vi "output.vi"(8 "error in":errorcluster, 10 "data table in":T1, 11 "dds runtime in":refnum<class "dds runtime.lvclass">) -> (0 "error out":errorcluster, 2 "data table out":T1, 3 "dds runtime out":refnum<class "dds runtime.lvclass">)   [LabVIEW 2015, in "DDS runtime.lvclass"]
doc: "Provides an interface for writing data to a module at runtime. While this interface performs no operations, a child should provide an override which may write to any open sessions, references, or interfaces."
uses:
  DDS runtime.lvclass
  <vilib>/NI/Tag Bus/table/data table.ctl
  DDS runtime.lvclass/dds runtime.ctl
  <vilib>/NI/Tag Bus/table/data polymorphs/read one/read Double.vi
  <vilib>/RTI DDS Toolkit/VIs/Write_Num.vi
  <vilib>/NI/Tag Bus/table/data polymorphs/read one/read Single.vi
  <vilib>/RTI DDS Toolkit/VIs/Write_NumSgl.vi
  <vilib>/NI/Tag Bus/table/data polymorphs/read one/read I64.vi
  <vilib>/RTI DDS Toolkit/VIs/Write_NumI64.vi
  <vilib>/NI/Tag Bus/table/data polymorphs/read one/read I32.vi
  <vilib>/RTI DDS Toolkit/VIs/Write_NumI32.vi
  <vilib>/NI/Tag Bus/table/data polymorphs/read one/read I16.vi
  <vilib>/RTI DDS Toolkit/VIs/Write_NumI16.vi
  <vilib>/NI/Tag Bus/table/data polymorphs/read one/read I8.vi
  <vilib>/RTI DDS Toolkit/VIs/Write_NumI8.vi
  <vilib>/NI/Tag Bus/table/data polymorphs/read one/read U64.vi
  <vilib>/RTI DDS Toolkit/VIs/Write_NumU64.vi
  <vilib>/NI/Tag Bus/table/data polymorphs/read one/read U32.vi
  <vilib>/RTI DDS Toolkit/VIs/Write_NumU32.vi
  <vilib>/NI/Tag Bus/table/data polymorphs/read one/read U16.vi
  <vilib>/RTI DDS Toolkit/VIs/Write_NumU16.vi
  <vilib>/NI/Tag Bus/table/data polymorphs/read one/read U8.vi
  <vilib>/RTI DDS Toolkit/VIs/Write_NumU8.vi
  <vilib>/NI/Tag Bus/table/data polymorphs/read one/read Boolean.vi
  <vilib>/RTI DDS Toolkit/VIs/Write_Bool.vi
  <vilib>/NI/Tag Bus/table/data polymorphs/read one/read String.vi
  <vilib>/RTI DDS Toolkit/VIs/Write_String.vi
  <vilib>/RTI DDS Toolkit/Library/LVDDS_library.lvlib
  <vilib>/NI/Tag Bus/table/data table.lvlib
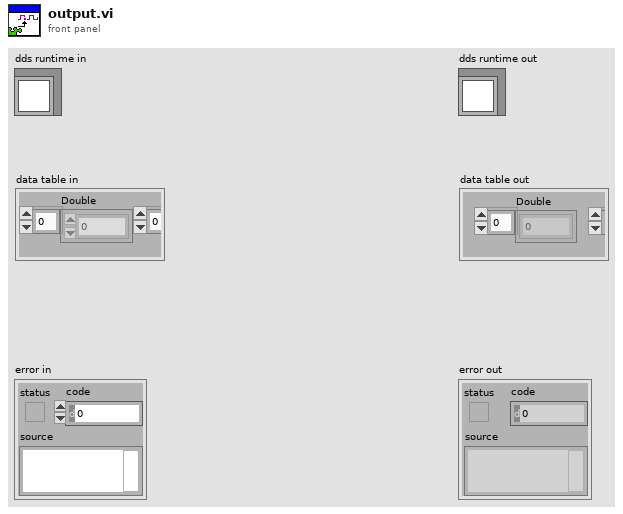
[diagram p1: front panel]
types:
  T1 = typedef "tag bus.lvlib/data table.lvlib/data table.ctl" = cluster{"Double":dbl[], "Single":sgl[], "I64":i64[], "I32":i32[], "I16":i16[], "I8":i8[], "U64":u64[], "U32":u32[], "U16":u16[], "U8":u8[], "Boolean":bool[], "String":string[], "Array of Double":cluster{"DBL Array":dbl[]}[], "Array of Single":cluster{"SGL Array":sgl[]}[], "Array of I64":cluster{"I64 Array":i64[]}[], "Array of I32":cluster{"I32 Array":i32[]}[], "Array of I16":cluster{"I16 Array":i16[]}[], "Array of I8":cluster{"I8 Array":i8[]}[], "Array of U64":cluster{"U64 Array":u64[]}[], "Array of U32":cluster{"U32 Array":u32[]}[], "Array of U16":cluster{"U16 Array":u16[]}[], "Array of U8":cluster{"U8 Array":u8[]}[], "Array of Boolean":cluster{"Boolean Array":bool[]}[], "Array of String":cluster{"String Array":string[]}[]}
  T2 = typedef "tag bus.lvlib/tag descriptor.lvclass/Data Type.ctl" = enum16{"Double", "Single", "I64", "I32", "I16", "I8", "U64", "U32", "U16", "U8", "Boolean", "String", "Array of Double", "Array of Single", "Array of I64", "Array of I32", "Array of I16", "Array of I8", "Array of U64", "Array of U32", "Array of U16", "Array of U8", "Array of Boolean", "Array of String"}
  T3 = cluster{"index":i32, "data type":T2, "ref num":u64}[]
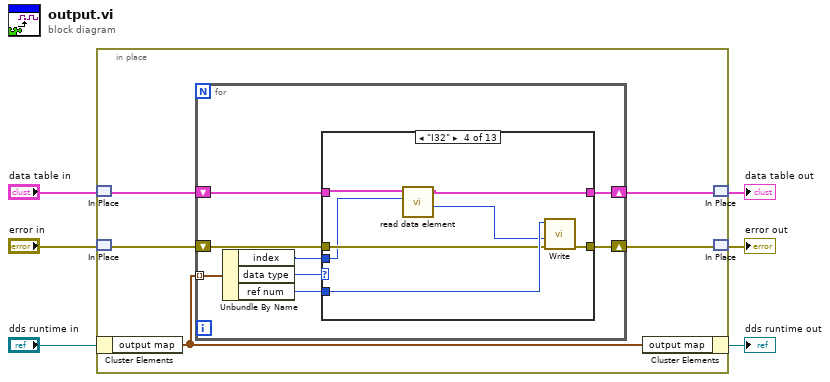
[diagram p0: block diagram]
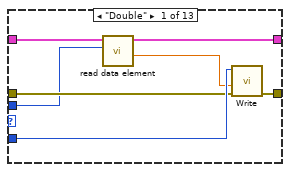
[diagram p2: hidden frame]
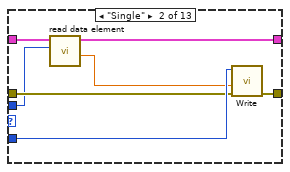
[diagram p3: hidden frame]
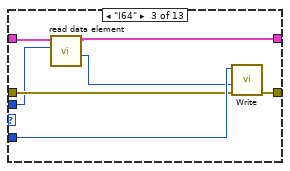
[diagram p4: hidden frame]
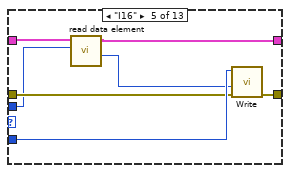
[diagram p5: hidden frame]
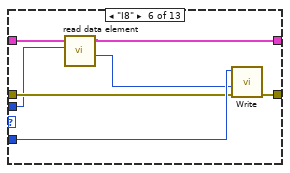
[diagram p6: hidden frame]
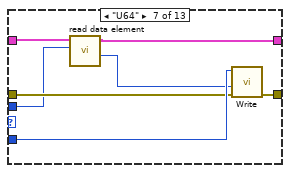
[diagram p7: hidden frame]
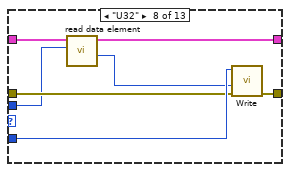
[diagram p8: hidden frame]
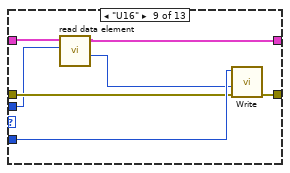
[diagram p9: hidden frame]
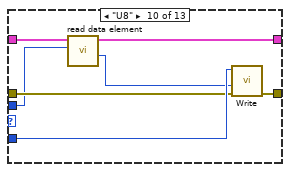
[diagram p10: hidden frame]
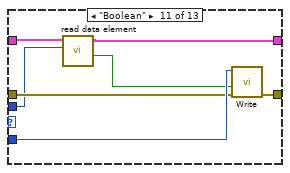
[diagram p11: hidden frame]
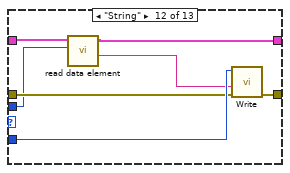
[diagram p12: hidden frame]
diagram:
  n1 = in-place {
    n2 = in-place-match #1("data table in") -> (w11:T1)
    n3 = in-place-match #2("error in") -> (w10:errorcluster)
    n4 = in-place-cluster #3("dds runtime in") -> ("output map"=w7:T3)
    n5 = for {
      tunnel: w7 -> [w19] mode=indexing
      shift-right: [w13] -> w8
      shift-left: w11 -> [w18]
      shift-right: [w14] -> w9
      shift-left: w10 -> [w15]
      n6 = Unbundle By Name(w19) -> ("index"=w17:i32, "data type"=w12:T2, "ref num"=w16:u64)
      n7 = case shown="\"I32\"" w12 {
        tunnel: w18 -> [w21 w30 w37 w44 w51 w58 w65 w72 w78 w86 w93 w100 w105]
        tunnel: w17 -> [w20 w28 w35 w41 w48 w56 w62 w69 w77 w83 w90 w98 _]
        tunnel: w16 -> [w26 w33 w40 w47 w54 w61 w68 w75 w82 w89 w96 w103 _]
        tunnel: w15 -> [w24 w32 w39 w46 w53 w60 w67 w74 w81 w88 w95 w102 w104]
        tunnel: [w23 w31 w38 w45 w52 w59 w66 w73 w80 w87 w94 w101 w104] -> w14
        tunnel: [w22 w29 w36 w43 w50 w57 w64 w71 w79 w85 w92 w99 w105] -> w13
        frame "Double" {
          n8 = call-poly <vilib>:"read data element.vi"("index"=w20, "data table in"=w21) -> ("value"=w25:dbl, "data table out"=w22:T1)  [unwired: 8 in]
          n9 = call-poly <vilib>:"Write.vi"("error in (no error)"=w24, "Data"=w25, "DDS Object Ref in"=w26) -> ("error out"=w23:errorcluster)  [unwired: 7 in, 1 out]
        }
        frame "Single" {
          n10 = call-poly <vilib>:"read data element.vi"("index"=w28, "data table in"=w30) -> ("value"=w27:sgl, "data table out"=w29:T1)  [unwired: 8 in]
          n11 = call-poly <vilib>:"Write.vi"("error in (no error)"=w32, "Data"=w27, "DDS Object Ref in"=w33) -> ("error out"=w31:errorcluster)  [unwired: 7 in, 1 out]
        }
        frame "I64" {
          n12 = call-poly <vilib>:"read data element.vi"("index"=w35, "data table in"=w37) -> ("value"=w34:i64, "data table out"=w36:T1)  [unwired: 8 in]
          n13 = call-poly <vilib>:"Write.vi"("error in (no error)"=w39, "Data"=w34, "DDS Object Ref in"=w40) -> ("error out"=w38:errorcluster)  [unwired: 7 in, 1 out]
        }
        frame "I32" {
          n14 = call-poly <vilib>:"read data element.vi"("index"=w41, "data table in"=w44) -> ("value"=w42:i32, "data table out"=w43:T1)  [unwired: 8 in]
          n15 = call-poly <vilib>:"Write.vi"("error in (no error)"=w46, "Data"=w42, "DDS Object Ref in"=w47) -> ("error out"=w45:errorcluster)  [unwired: 7 in, 1 out]
        }
        frame "I16" {
          n16 = call-poly <vilib>:"read data element.vi"("index"=w48, "data table in"=w51) -> ("value"=w49:i16, "data table out"=w50:T1)  [unwired: 8 in]
          n17 = call-poly <vilib>:"Write.vi"("error in (no error)"=w53, "Data"=w49, "DDS Object Ref in"=w54) -> ("error out"=w52:errorcluster)  [unwired: 7 in, 1 out]
        }
        frame "I8" {
          n18 = call-poly <vilib>:"read data element.vi"("index"=w56, "data table in"=w58) -> ("value"=w55:i8, "data table out"=w57:T1)  [unwired: 8 in]
          n19 = call-poly <vilib>:"Write.vi"("error in (no error)"=w60, "Data"=w55, "DDS Object Ref in"=w61) -> ("error out"=w59:errorcluster)  [unwired: 7 in, 1 out]
        }
        frame "U64" {
          n20 = call-poly <vilib>:"read data element.vi"("index"=w62, "data table in"=w65) -> ("value"=w63:u64, "data table out"=w64:T1)  [unwired: 8 in]
          n21 = call-poly <vilib>:"Write.vi"("error in (no error)"=w67, "Data"=w63, "DDS Object Ref in"=w68) -> ("error out"=w66:errorcluster)  [unwired: 7 in, 1 out]
        }
        frame "U32" {
          n22 = call-poly <vilib>:"read data element.vi"("index"=w69, "data table in"=w72) -> ("value"=w70:u32, "data table out"=w71:T1)  [unwired: 8 in]
          n23 = call-poly <vilib>:"Write.vi"("error in"=w74, "Data"=w70, "DDS Object Ref in"=w75) -> ("error out"=w73:errorcluster)  [unwired: 7 in, 1 out]
        }
        frame "U16" {
          n24 = call-poly <vilib>:"read data element.vi"("index"=w77, "data table in"=w78) -> ("value"=w76:u16, "data table out"=w79:T1)  [unwired: 8 in]
          n25 = call-poly <vilib>:"Write.vi"("error in (no error)"=w81, "Data"=w76, "DDS Object Ref in"=w82) -> ("error out"=w80:errorcluster)  [unwired: 7 in, 1 out]
        }
        frame "U8" {
          n26 = call-poly <vilib>:"read data element.vi"("index"=w83, "data table in"=w86) -> ("value"=w84:u8, "data table out"=w85:T1)  [unwired: 8 in]
          n27 = call-poly <vilib>:"Write.vi"("error in"=w88, "Data"=w84, "DDS Object Ref in"=w89) -> ("error out"=w87:errorcluster)  [unwired: 7 in, 1 out]
        }
        frame "Boolean" {
          n28 = call-poly <vilib>:"read data element.vi"("index"=w90, "data table in"=w93) -> ("value"=w91:bool, "data table out"=w92:T1)  [unwired: 8 in]
          n29 = call-poly <vilib>:"Write.vi"("error in (no error)"=w95, "Data"=w91, "DDS Object Ref in"=w96) -> ("error out"=w94:errorcluster)  [unwired: 7 in, 1 out]
        }
        frame "String" {
          n30 = call-poly <vilib>:"read data element.vi"("index"=w98, "data table in"=w100) -> ("value"=w97:string, "data table out"=w99:T1)  [unwired: 8 in]
          n31 = call-poly <vilib>:"Write.vi"("error in (no error)"=w102, "Data"=w97, "DDS Object Ref in"=w103) -> ("error out"=w101:errorcluster)  [unwired: 7 in, 1 out]
        }
        frame Default {
          # "#TODO:\nThis case should never be reached.\nThrow an error."
        }
      }
    }
    n32 = in-place-cluster #3("output map"=w7) -> (→"dds runtime out":refnum<class "dds runtime.lvclass">)
    n33 = in-place-match #1(w8) -> (→"data table out":T1)
    n34 = in-place-match #2(w9) -> (→"error out":errorcluster)
  }
